vi "execute_value_write_policy.vi"(8 "error in (no error)":errorcluster, 9 "Publish Time":timestamp, 10 "New Topic Value":variant, 11 "TriggeredSubscription In":refnum<class "TriggeredSubscription.lvclass">) -> (0 "error out":errorcluster, 3 "TriggeredSubscription Out":refnum<class "TriggeredSubscription.lvclass">)   [LabVIEW 2015, in "SubscriptionPolicy.lvlib" / "TriggeredSubscription.lvclass"]
uses:
  TriggeredSubscription.lvclass
  TriggeredSubscription.lvclass/TriggeredSubscription.ctl
  IMediator/ISubscriptionPolicy/ISubscriptionPolicy.lvclass/ISubscriptionPolicy.ctl
  <vilib>/Utility/error.llb/Error Cluster From Error Code.vi
  <vilib>/ErrorRing/Error Ring.xnode
  IMediator/ITransport/ITransport.lvclass
  IMediator/ISubscriptionPolicy/ISubscriptionPolicy.lvclass
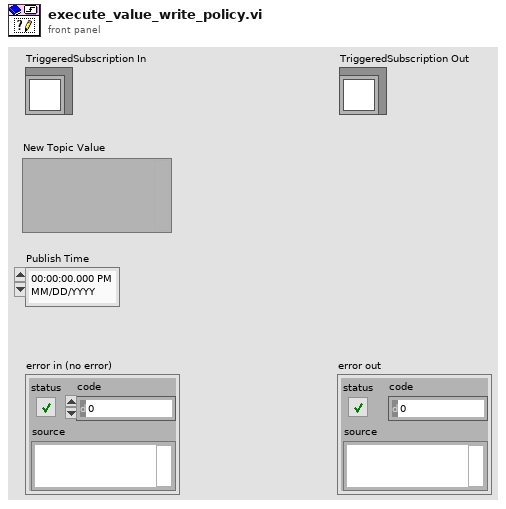
[diagram p1: front panel]
types:
  T1 = enum16{"Equal", "Not equal", "Greater than", "Less than", "Greater or equal", "Less or equal"}
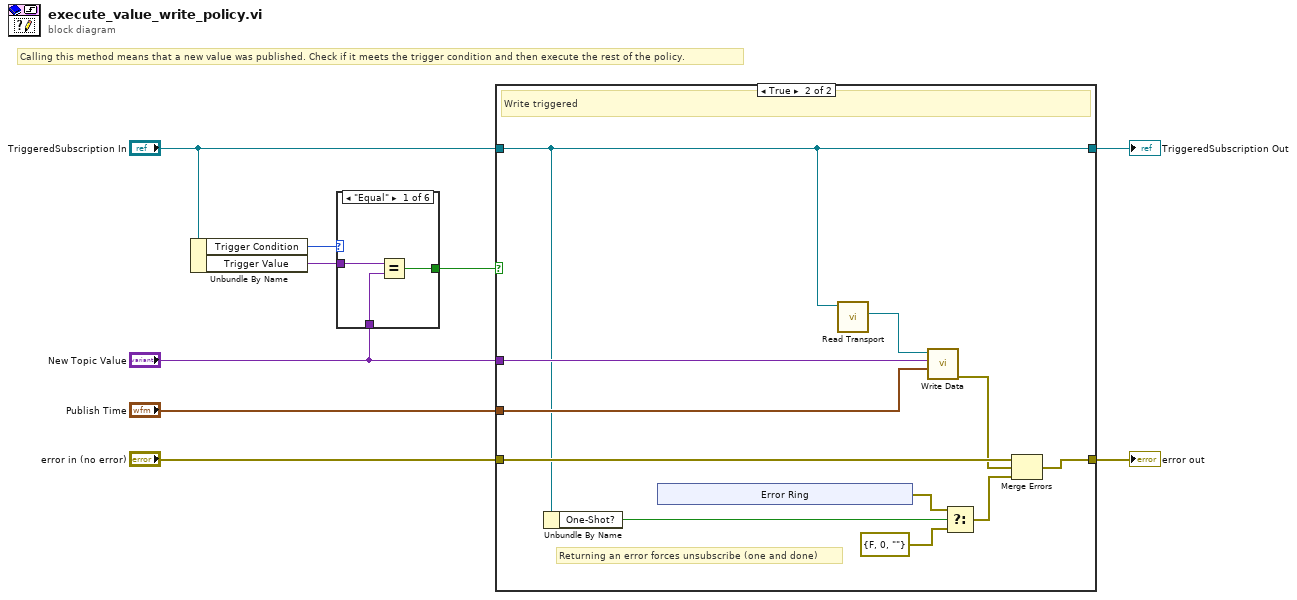
[diagram p0: block diagram]
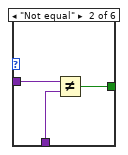
[diagram p3: hidden frame]
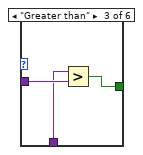
[diagram p4: hidden frame]
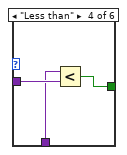
[diagram p5: hidden frame]
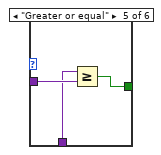
[diagram p6: hidden frame]
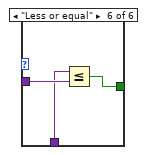
[diagram p7: hidden frame]
diagram:
  # "Calling this method means that a new value was published. Check if it meets the trigger condition and then execute the rest of the policy."
  n1 = Unbundle By Name("TriggeredSubscription In") -> ("Trigger Condition"=w5:T1, "Trigger Value"=w4:variant)
  n2 = case shown="\"Equal\"" w5 {
    tunnel: w4 -> [w12 w15 w18 w21 w24 w27]
    tunnel: "New Topic Value" -> [w11 w14 w17 w20 w23 w26]
    tunnel: [w10 w13 w16 w19 w22 w25] -> w1
    frame "Equal" {
      n3 = Equal?(x=w12, y=w11) -> (x = y?=w10:bool)
    }
    frame "Not equal" {
      n4 = Not Equal?(x=w15, y=w14) -> (x != y?=w13:bool)
    }
    frame "Greater than" {
      n5 = Greater?(x=w17, y=w18) -> (0:w16:bool)
    }
    frame "Less than" {
      n6 = Less?(x=w20, y=w21) -> (x < y?=w19:bool)
    }
    frame "Greater or equal" {
      n7 = Greater Or Equal?(x=w23, y=w24) -> (x >= y?=w22:bool)
    }
    frame "Less or equal" {
      n8 = Less Or Equal?(x=w26, y=w27) -> (x <= y?=w25:bool)
    }
  }
  n9 = case shown="True" w1 {
    tunnel: "Publish Time" -> [_ w40]
    tunnel: "error in (no error)" -> [w28 w39]
    tunnel: [w28 w38] -> w7
    tunnel: "TriggeredSubscription In" -> [w29 w34]
    tunnel: "New Topic Value" -> [_ w35]
    tunnel: [w29 w34] -> w2
    frame False {
      # "Write NOT triggered"
    }
    frame True {
      # "Returning an error forces unsubscribe (one and done)"
      # "Write triggered"
      n10 = Unbundle By Name(w34) -> ("One-Shot?"=w33:bool)
      n11 = xnode "Error Ring"() -> ("error out"=w31:errorcluster)
      n12 = call "Read Transport.vi"("ISubscriptionPolicy in"=w34) -> ("Transport"=w36:refnum<class "ITransport.lvclass">)  [unwired: 10 in]
      n13 = call-dynamic "Write Data.vi"("Publication Time"=w40, "Value"=w35, "ITransport in"=w36) -> ("error out"=w37:errorcluster)  [unwired: 7 in, 1 out]
      n14 = Select(t=w31, s=w33, f=errorcluster {"status"=FALSE, "code"=0, "source"=""}) -> (s? t:f=w32:errorcluster)
      n15 = Merge Errors(w39, w37, w32) -> (w38:errorcluster)
    }
  }
  "error out" <- w7
  "TriggeredSubscription Out" <- w2
